vi "filter_logic_delays_test.vi"() -> ()   [LabVIEW 2015]
uses:
  <vilib>/Platform/TimedLoop/XDataNode/timing_clust.ctl
  <vilib>/Platform/TimedLoop/XDataNode/nitl_modes.ctl
  <vilib>/Platform/TimedLoop/XDataNode/wakeup.ctl
  <vilib>/rvi/Emulation/niFpgaGetClockAttributes.vi
  <vilib>/rvi/Emulation/niFpgaSctlEmulationGetInTimedLoop.vi
  <vilib>/rvi/Emulation/niFpgaEmulationReportErrorSimple.vi
  <vilib>/rvi/Emulation/niFpgaProcessEmulError.vi
  <vilib>/rvi/eio/common/nirviEmuTemplateMethod_errors.vi
  <vilib>/rvi/Emulation/niFpgaCriticalErrorInLSC.vi
  <vilib>/eio/EIONode/EIONode.xnode
  <vilib>/Platform/TimedLoop/XDataNode/XDataNode.xnode
  <vilib>/Platform/TimedLoop/XDataNode/XDNodeRunTimeDep.lvlib
panel:
  in  "One Shot":bool
  in  "High Charge Limit":i16
  in  "Low Charge Limit":i16
  in  "High Velocity Count":i32
  in  "Low Velocity Count":i32
  in  "High Mass Limit":i64
  in  "Low Mass Limit":i64
  in  "Mult1":fxp<+,16,7>
  out "Plates":bool
  out "Delay":bool
  out "Armed":bool
  out "Del Armed":bool
  in  "Reset One Shot":bool
  in  "Filter threshold 1":i32=1000
  in  "Filter threshold 2":i32=1000
  in  "Filter threshold 3":i32=1000
  in  "Filter threshold 4":i32=1000
  in  "Filter threshold 5":i32=1000
  in  "Filter threshold 6":i32=1000
  in  "Filter threshold 7":i32=1000
  out "Detector 1 Correlation 2":i16
  out "Detector 1 Correlation 1":i16
  out "Detector 3 Correlation 1":i16
  out "Detector 3 Correlation 2":i16
  out "Detector 1 Correlation 3":i16
  out "Detector 1 Correlation 4":i16
  out "Detector 3 Correlation 3":i16
  out "Detector 1 Correlation 5":i16
  out "Detector 3 Correlation 4":i16
  out "Detector 1 Correlation 6":i16
  out "Detector 3 Correlation 5":i16
  out "Detector 1 Correlation 7":i16
  out "Detector 3 Correlation 6":i16
  out "Detector 3 Correlation 7":i16
  out "IO Module\\AI 0":i16
  out "IO Module\\AI 1":i16
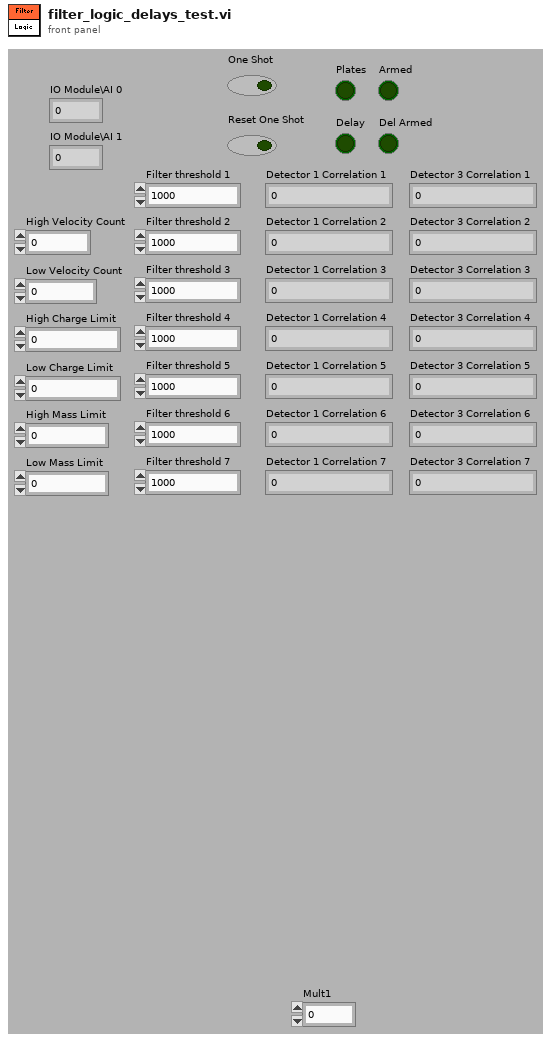
[diagram p1: front panel]
types:
  T1 = typedef "XDNodeRunTimeDep.lvlib/timing_clust.ctl" = cluster{"Expected End [f-1]":u64, "Actual End [f-1]":u64, "Finished Late? [f-1]":bool, "Expected End [i-1]":u64, "Actual End [i-1]":u64, "Finished Late? [i-1]":bool, "Expected Start [i]":u64, "Actual Start [i]":u64, "Expected Start [f]":u64, "Actual Start [f]":u64, "Source Name":string, "Structure Name":string, "Period":i64, "Deadline":i64, "Offset":i64, "Start":i64, "Priority":i32, "Timeout":i32, "Mode":T2, "Wakeup Reason":T3, "Error":errorcluster, "Source Type":string, "Secondary Source Type":string, "Global End Time":u64, "Global Start Time":u64, "Frame Duration":u64, "Iteration Duration":u64, "Assigned CPU":i32, "I/O Scan Engine Mode":u32}
  T2 = typedef "XDNodeRunTimeDep.lvlib/nitl_modes.ctl" = enum32{"No Change", "Process missed periods, maintain original phase", "Discard missed periods, maintain original phase", "Process missed periods, ignore original phase", "Discard missed periods, ignore original phase"}
  T3 = typedef "XDNodeRunTimeDep.lvlib/wakeup.ctl" = enum32{"Normal", "Aborted", "Asynchronous wakeup", "Timing source error", "Timed loop error", "Timeout"}
  T4 = typedef "Limits.ctl" = cluster{"High Charge Limit":i16, "Low Charge Limit":i16, "Time Out Limit":i32, "High Velocity Count":i32, "Low Velocity Count":i32, "Sampling Rate":fxp<+,30,25>, "High Mass Limit":i64, "Low Mass Limit":i64}
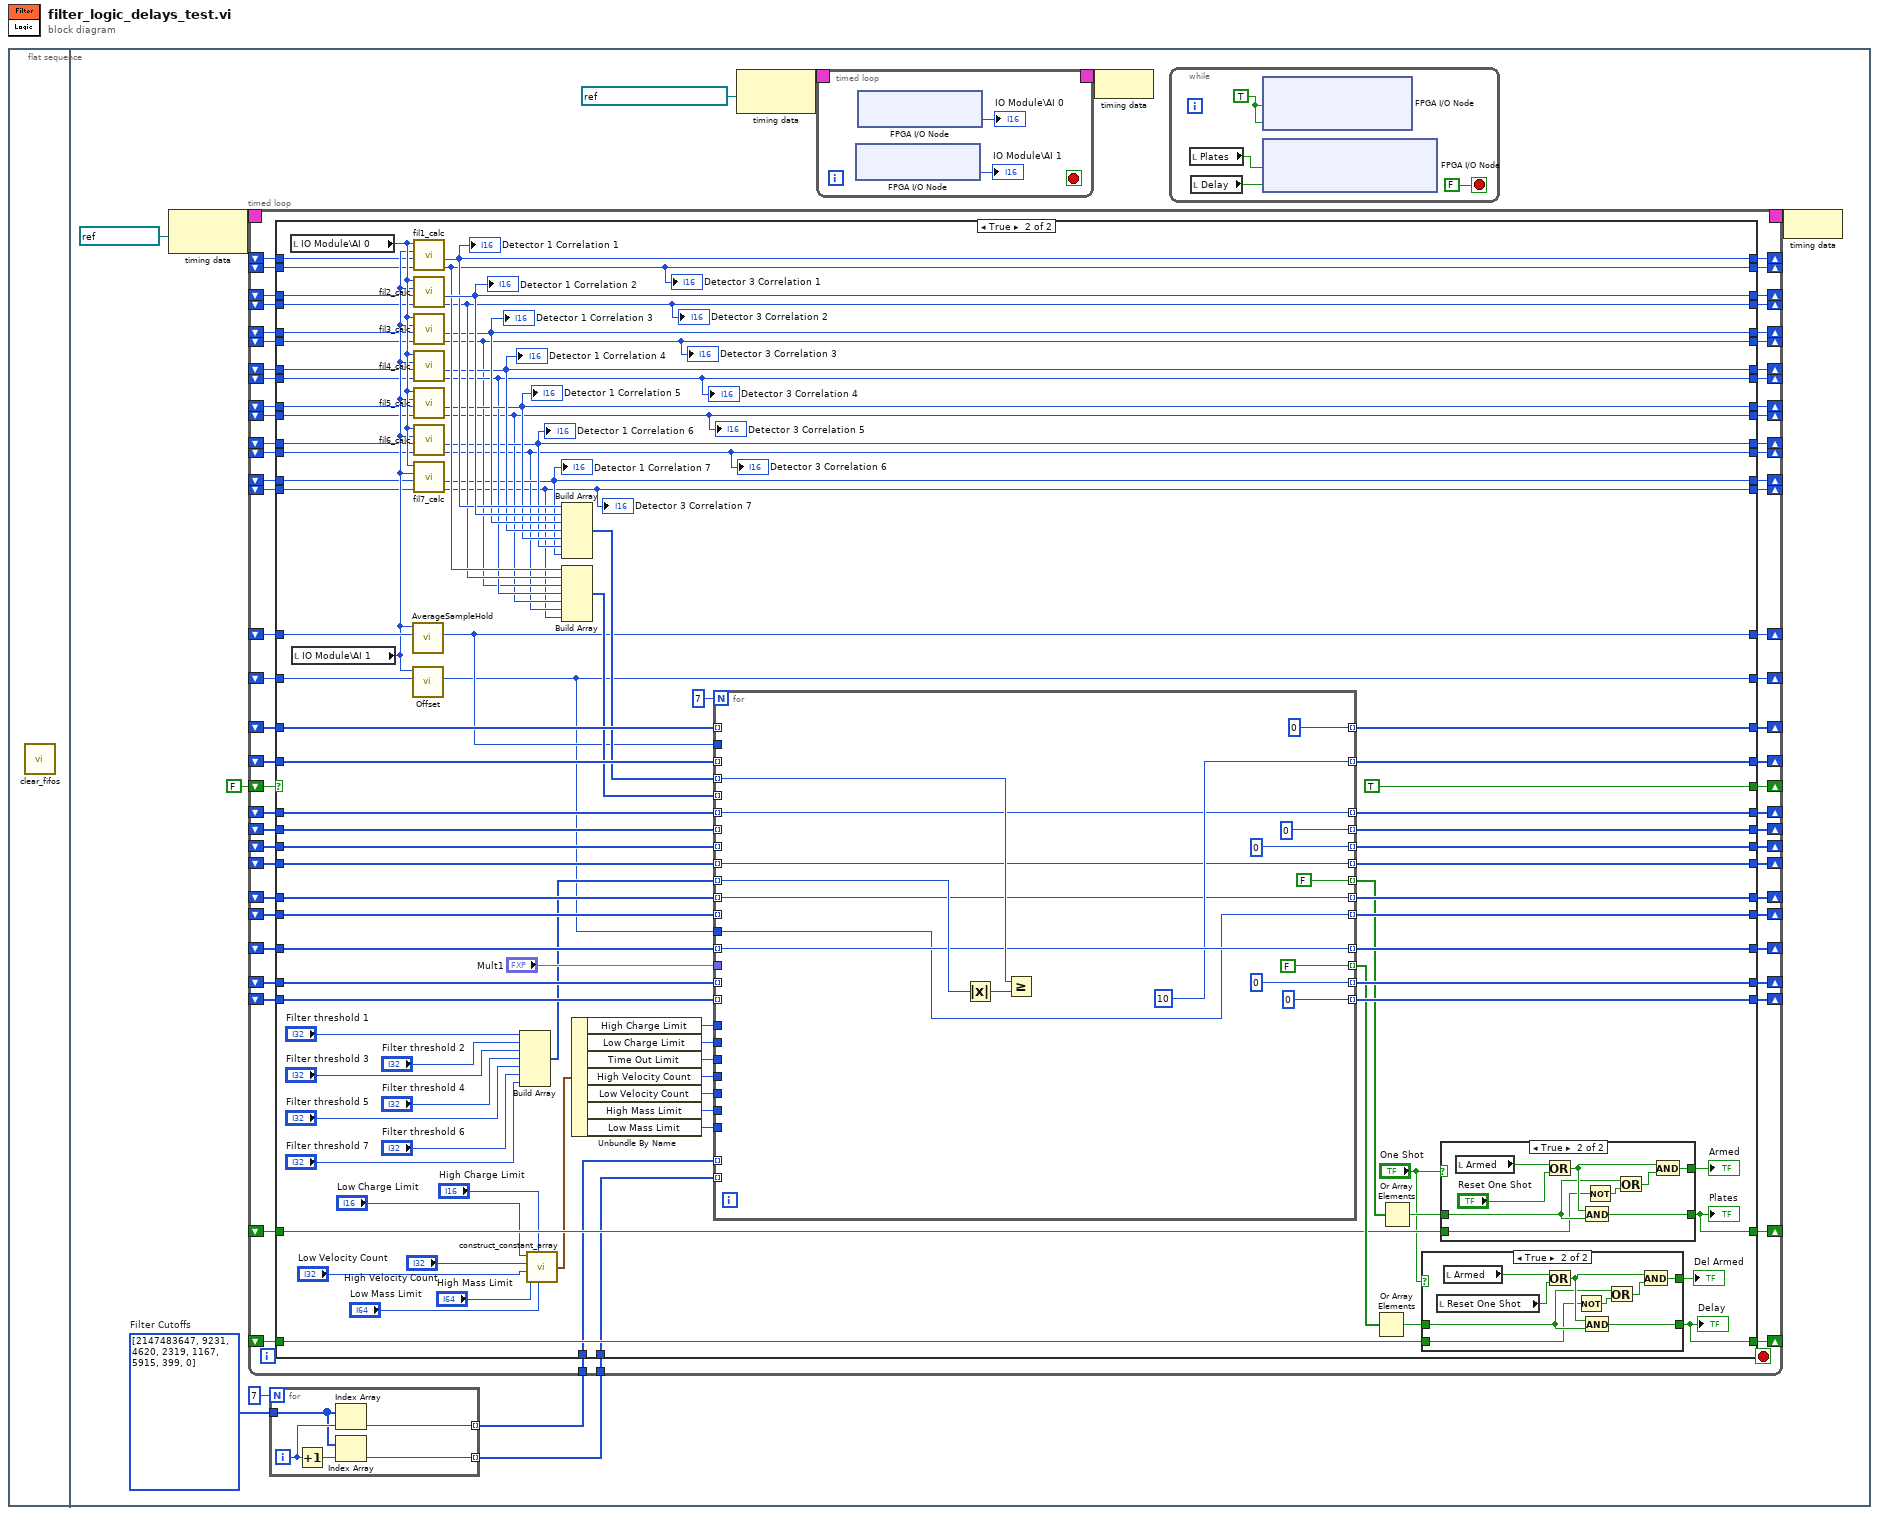
[diagram p0: block diagram]
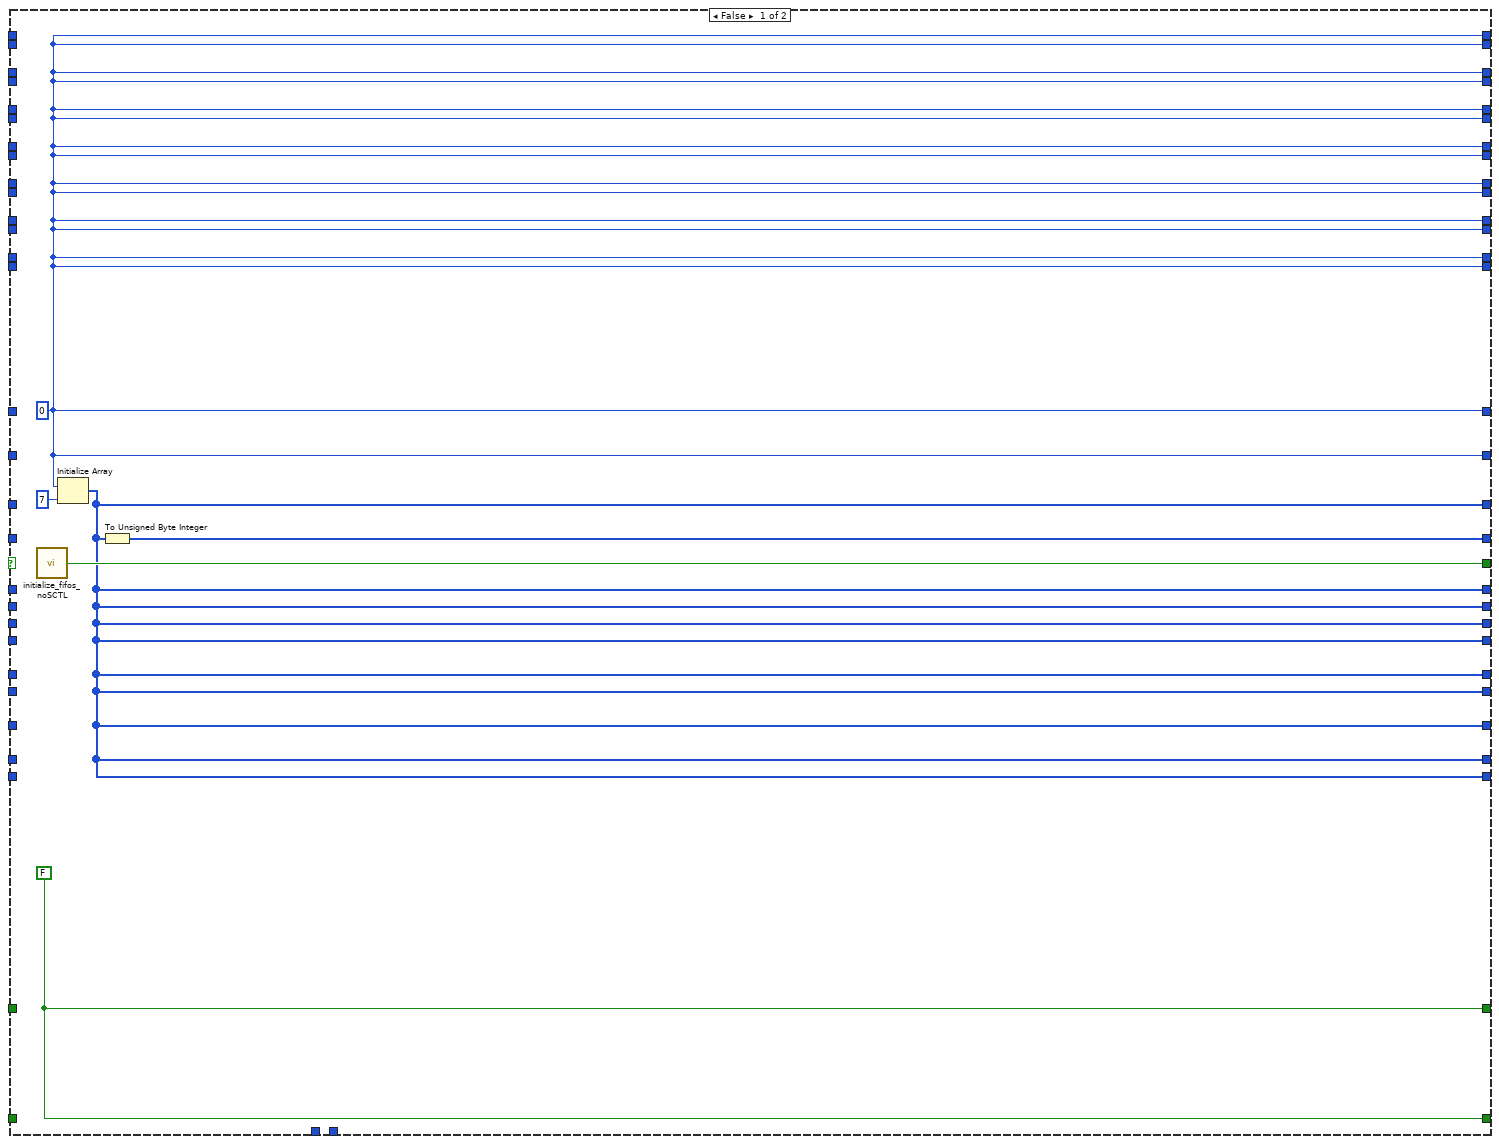
[diagram p2: hidden frame]
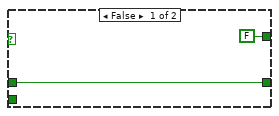
[diagram p3: hidden frame]
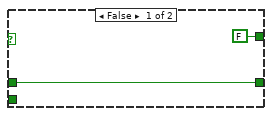
[diagram p4: hidden frame]
diagram:
  n1 = flat-sequence {
    frame #0 {
      n2 = call "clear_fifos.vi"() -> ()  [unwired: 1 in]
    }
    frame #1 {
      w3 = i32[] [2147483647, 9231, 4620, 2319, 1167, 5915, 399, 0]  # Filter Cutoffs
      n3 = node-c288(refnum<k21> "26.67MHz" ("Source Name")) -> (w11:T1)
      n4 = for {
        N: 7 -> [_]
        tunnel: w3 -> [w14]
        tunnel: [w13] -> w2 mode=indexing
        tunnel: [w12] -> w1 mode=indexing
        i -> [w16]
        n5 = Increment(x=w16) -> (x+1=w15:i32)
        n6 = Index Array(array=w14, index=w16) -> (element=w13:i32)
        n7 = Index Array(array=w14, index=w15) -> (element=w12:i32)
      }
      n8 = timed-loop {
        timing: w11 -> [_]
        timing-out: [_] -> w10
        shift-right: [w89] -> _
        shift-left: FALSE -> [w90]
        shift-right: [w87] -> _
        shift-left: _ -> [w88]
        shift-right: [w85] -> _
        shift-left: _ -> [w86]
        shift-right: [w83] -> _
        shift-left: _ -> [w84]
        shift-right: [w69] -> _
        shift-left: _ -> [w82]
        shift-right: [w80] -> _
        shift-left: _ -> [w81]
        shift-right: [w78] -> _
        shift-left: _ -> [w79]
        shift-right: [w68] -> _
        shift-left: _ -> [w77]
        shift-right: [w67] -> _
        shift-left: _ -> [w76]
        shift-right: [w63] -> _
        shift-left: _ -> [w75]
        shift-right: [w73] -> _
        shift-left: _ -> [w74]
        shift-right: [w66] -> _
        shift-left: _ -> [w72]
        shift-right: [w65] -> _
        shift-left: _ -> [w71]
        shift-right: [w64] -> _
        shift-left: _ -> [w70]
        shift-right: [w62] -> _
        shift-left: _ -> [w61]
        shift-right: [w59] -> _
        shift-left: _ -> [w60]
        shift-right: [w58] -> _
        shift-left: _ -> [w57]
        shift-right: [w56] -> _
        shift-left: _ -> [w55]
        shift-right: [w54] -> _
        shift-left: _ -> [w50]
        shift-right: [w53] -> _
        shift-left: _ -> [w49]
        shift-right: [w52] -> _
        shift-left: _ -> [w48]
        shift-right: [w51] -> _
        shift-left: _ -> [w47]
        shift-right: [w46] -> _
        shift-left: _ -> [w38]
        shift-right: [w45] -> _
        shift-left: _ -> [w37]
        shift-right: [w44] -> _
        shift-left: _ -> [w36]
        shift-right: [w43] -> _
        shift-left: _ -> [w31]
        shift-right: [w42] -> _
        shift-left: _ -> [w35]
        shift-right: [w41] -> _
        shift-left: _ -> [w32]
        shift-right: [w40] -> _
        shift-left: _ -> [w34]
        shift-right: [w39] -> _
        shift-left: _ -> [w33]
        tunnel: w2 -> [w30]
        tunnel: w1 -> [w29]
        stop <- _ stop-if-true
        n9 = case shown="True" w90 {
          tunnel: [w96 TRUE] -> w89
          tunnel: w88 -> [_ w191]
          tunnel: [w93 w190] -> w87
          tunnel: w86 -> [_ w189]
          tunnel: [w91 w123] -> w85
          tunnel: w84 -> [_ w188]
          tunnel: [w94 w187] -> w83
          tunnel: w82 -> [_ w186]
          tunnel: w81 -> [_ w185]
          tunnel: [w93 w184] -> w80
          tunnel: w79 -> [_ w183]
          tunnel: [w93 w182] -> w78
          tunnel: w77 -> [_ w181]
          tunnel: w76 -> [_ w180]
          tunnel: w75 -> [_ w179]
          tunnel: w74 -> [_ w178]
          tunnel: [w91 w122] -> w73
          tunnel: w72 -> [_ w177]
          tunnel: w71 -> [_ w176]
          tunnel: w70 -> [_ w175]
          tunnel: [w93 w174] -> w69
          tunnel: [w93 w173] -> w68
          tunnel: [w93 w172] -> w67
          tunnel: [w93 w171] -> w66
          tunnel: [w93 w170] -> w65
          tunnel: [w93 w169] -> w64
          tunnel: [w93 w168] -> w63
          tunnel: [w95 w162] -> w62
          tunnel: w61 -> [_ w163]
          tunnel: w60 -> [_ w159]
          tunnel: [w95 w158] -> w59
          tunnel: [w91 w108] -> w58
          tunnel: w57 -> [_ w137]
          tunnel: [w91 w110] -> w56
          tunnel: w55 -> [_ w136]
          tunnel: [w91 w109] -> w54
          tunnel: [w91 w112] -> w53
          tunnel: [w91 w111] -> w52
          tunnel: [w91 w115] -> w51
          tunnel: w50 -> [_ w135]
          tunnel: w49 -> [_ w134]
          tunnel: w48 -> [_ w133]
          tunnel: w47 -> [_ w132]
          tunnel: [w91 w114] -> w46
          tunnel: [w91 w116] -> w45
          tunnel: [w91 w113] -> w44
          tunnel: [w91 w117] -> w43
          tunnel: [w91 w118] -> w42
          tunnel: [w91 w121] -> w41
          tunnel: [w91 w119] -> w40
          tunnel: [w91 w120] -> w39
          tunnel: w38 -> [_ w131]
          tunnel: w37 -> [_ w130]
          tunnel: w36 -> [_ w129]
          tunnel: w35 -> [_ w128]
          tunnel: w34 -> [_ w127]
          tunnel: w33 -> [_ w126]
          tunnel: w32 -> [_ w125]
          tunnel: w31 -> [_ w124]
          tunnel: w30 -> [_ w107]
          tunnel: w29 -> [_ w106]
          frame False {
            w95 = FALSE
            w91 = i16 0 ("Output New Average")
            n10 = call "initialize_fifos_noSCTL.vi"() -> ("Output State"=w96:bool)
            n11 = Initialize Array(w91, 7 ("dimension size")) -> (w93:i16[])
            n12 = To Unsigned Byte Integer(number=w93) -> (unsigned 8bit integer=w94:u8[])
          }
          frame True {
            n13 = local read "IO Module\\AI 0"() -> (w149:i16)
            n14 = local read "IO Module\\AI 1"() -> (w148:i16)
            n15 = call "AverageSampleHold.vi"("Previous Average"=w189, "Input Value"=w148) -> ("Output New Average"=w123:i16)  [unwired: 9 in]
            n16 = call "Offset.vi"("Previous Average"=w178, "Input Value"=w148) -> ("Output New Average"=w122:i16)  [unwired: 9 in]
            n17 = call "fil1_calc.vi"("Detector 3 Correlation In"=w127, "Detector 1 Correlation In"=w126, "AI1"=w148, "AI0"=w149) -> ("Detector 3 Correlation Out"=w119:i16, "Detector 1 Correlation Out"=w120:i16)  [unwired: 4 in]
            "Detector 1 Correlation 1" <- w120
            "Detector 3 Correlation 1" <- w119
            n18 = call "fil2_calc.vi"("Detector 3 Correlation In"=w128, "Detector 1 Correlation In"=w125, "AI1"=w148, "AI0"=w149) -> ("Detector 3 Correlation Out"=w118:i16, "Detector 1 Correlation Out"=w121:i16)  [unwired: 4 in]
            "Detector 1 Correlation 2" <- w121
            "Detector 3 Correlation 2" <- w118
            n19 = call "fil3_calc.vi"("Detector 3 Correlation In"=w129, "Detector 1 Correlation In"=w124, "AI1"=w148, "AI0"=w149) -> ("Detector 3 Correlation Out"=w113:i16, "Detector 1 Correlation Out"=w117:i16)  [unwired: 4 in]
            "Detector 1 Correlation 3" <- w117
            "Detector 3 Correlation 3" <- w113
            n20 = call "fil4_calc.vi"("Detector 3 Correlation In"=w131, "Detector 1 Correlation In"=w130, "AI1"=w148, "AI0"=w149) -> ("Detector 3 Correlation Out"=w114:i16, "Detector 1 Correlation Out"=w116:i16)  [unwired: 4 in]
            "Detector 1 Correlation 4" <- w116
            "Detector 3 Correlation 4" <- w114
            n21 = call "fil5_calc.vi"("Detector 3 Correlation In"=w133, "Detector 1 Correlation In"=w132, "AI1"=w148, "AI0"=w149) -> ("Detector 3 Correlation Out"=w111:i16, "Detector 1 Correlation Out"=w115:i16)  [unwired: 4 in]
            "Detector 1 Correlation 5" <- w115
            "Detector 3 Correlation 5" <- w111
            n22 = call "fil6_calc.vi"("Detector 3 Correlation In"=w135, "Detector 1 Correlation In"=w134, "AI1"=w148, "AI0"=w149) -> ("Detector 3 Correlation Out"=w109:i16, "Detector 1 Correlation Out"=w112:i16)  [unwired: 4 in]
            "Detector 1 Correlation 6" <- w112
            "Detector 3 Correlation 6" <- w109
            n23 = call "fil7_calc.vi"("Detector 3 Correlation In"=w137, "Detector 1 Correlation In"=w136, "AI1"=w148, "AI0"=w149) -> ("Detector 3 Correlation Out"=w108:i16, "Detector 1 Correlation Out"=w110:i16)  [unwired: 4 in]
            "Detector 1 Correlation 7" <- w110
            "Detector 3 Correlation 7" <- w108
            n24 = Build Array("Filter threshold 1", "Filter threshold 2", "Filter threshold 3", "Filter threshold 4", "Filter threshold 5", "Filter threshold 6", "Filter threshold 7") -> (w138:i32[])
            n25 = call "construct_constant_array.vi"("Low Mass Limit"="Low Mass Limit", "High Charge Limit"="High Charge Limit", "High Mass Limit"="High Mass Limit", "Low Velocity Count"="Low Velocity Count", "High Velocity Count"="High Velocity Count", "Low Charge Limit"="Low Charge Limit") -> ("Limits"=w105:T4)
            n26 = Build Array(w120, w121, w117, w116, w115, w112, w110) -> (w147:i16[])
            n27 = Build Array(w119, w118, w113, w114, w111, w109, w108) -> (w146:i16[])
            n28 = Unbundle By Name(w105) -> ("High Charge Limit"=w98:i16, "Low Charge Limit"=w99:i16, "Time Out Limit"=w100:i32, "High Velocity Count"=w101:i32, "Low Velocity Count"=w102:i32, "High Mass Limit"=w103:i64, "Low Mass Limit"=w104:i64)
            n29 = for {
              N: 7 -> [_]
              tunnel: w147 -> [w230] mode=indexing
              tunnel: w146 -> [_] mode=indexing
              tunnel: w191 -> [_] mode=indexing
              tunnel: [0 ("Old Average In")] -> w190 mode=indexing
              tunnel: w188 -> [_] mode=indexing
              tunnel: [u8 10] -> w187 mode=indexing
              tunnel: w186 -> [w225] mode=indexing
              tunnel: w185 -> [_] mode=indexing
              tunnel: [0] -> w184 mode=indexing
              tunnel: w183 -> [_] mode=indexing
              tunnel: [u16 0] -> w182 mode=indexing
              tunnel: w181 -> [_] mode=indexing
              tunnel: w180 -> [_] mode=indexing
              tunnel: w179 -> [w228] mode=indexing
              tunnel: w177 -> [w222] mode=indexing
              tunnel: w138 -> [w229] mode=indexing
              tunnel: w176 -> [w219] mode=indexing
              tunnel: w175 -> [_] mode=indexing
              tunnel: [w225] -> w174 mode=indexing
              tunnel: [0] -> w173 mode=indexing
              tunnel: [u32 0] -> w172 mode=indexing
              tunnel: [w222] -> w171 mode=indexing
              tunnel: [w219] -> w170 mode=indexing
              tunnel: [w218] -> w169 mode=indexing
              tunnel: [w228] -> w168 mode=indexing
              tunnel: [FALSE] -> w167 mode=indexing
              tunnel: [FALSE] -> w166 mode=indexing
              tunnel: "Mult1" -> [_]
              tunnel: w123 -> [_]
              tunnel: w122 -> [w218]
              tunnel: w107 -> [_] mode=indexing
              tunnel: w106 -> [_] mode=indexing
              tunnel: w104 -> [_]
              tunnel: w103 -> [_]
              tunnel: w102 -> [_]
              tunnel: w101 -> [_]
              tunnel: w100 -> [_]
              tunnel: w99 -> [_]
              tunnel: w98 -> [_]
              n30 = Absolute Value(x=w229) -> (abs(x)=w215:i32)
              n31 = Greater Or Equal?(x=w230, y=w215) -> ()  [unwired: 1 out]
            }
            n32 = Or Array Elements(Boolean array=w166) -> (logical OR=w161:bool)
            n33 = Or Array Elements(Boolean array=w167) -> (logical OR=w165:bool)
            n34 = case shown="True" "One Shot" {
              tunnel: [w194 w200] -> w158
              tunnel: w161 -> [w194 w197]
              tunnel: [FALSE w202] -> w157
              tunnel: w159 -> [_ w196]
              frame False {
              }
              frame True {
                n35 = local read "Reset One Shot"() -> (w195:bool)
                n36 = local read "Armed"() -> (w203:bool)
                n37 = Or(x=w203, y=w195) -> (x .or. y?=w201:bool)
                n38 = Not(x=w196) -> (.not. x?=w198:bool)
                n39 = And(x=w201, y=w197) -> (x .and. y?=w200:bool)
                n40 = Or(x=w197, y=w198) -> (x .or. y?=w199:bool)
                n41 = And(x=w201, y=w199) -> (x .and. y?=w202:bool)
              }
            }
            "Delay" <- w158
            "Del Armed" <- w157
            n42 = case shown="True" "One Shot" {
              tunnel: [w205 w210] -> w162
              tunnel: w165 -> [w205 w207]
              tunnel: [FALSE w212] -> w164
              tunnel: w163 -> [_ w206]
              frame False {
              }
              frame True {
                n43 = local read "Armed"() -> (w214:bool)
                n44 = Or(x=w214, y="Reset One Shot") -> (x .or. y?=w211:bool)
                n45 = And(x=w211, y=w207) -> (x .and. y?=w210:bool)
                n46 = Not(x=w206) -> (.not. x?=w208:bool)
                n47 = Or(x=w207, y=w208) -> (x .or. y?=w209:bool)
                n48 = And(x=w211, y=w209) -> (x .and. y?=w212:bool)
              }
            }
            "Plates" <- w162
            "Armed" <- w164
          }
        }
      }
      n49 = node-c288(refnum<k21> "IO Module\\Data Clock" ("Source Name")) -> (w8:T1)
      n50 = timed-loop {
        timing: w8 -> [_]
        timing-out: [_] -> w7
        stop <- _ stop-if-true
        n51 = xnode "FPGA I/O Node"() -> ("IO Module\\AI 1"=→"IO Module\\AI 1":i16)  [unwired: 1 in, 1 out]
        n52 = xnode "FPGA I/O Node"() -> ("IO Module\\AI 0"=→"IO Module\\AI 0":i16)  [unwired: 1 in, 1 out]
      }
      n53 = node-c288(w7) -> ()
      n54 = while {
        stop <- FALSE stop-if-true
        w28 = TRUE ("IO Module\\PFI Enable")
        n55 = local read "Plates"() -> (w26:bool)
        n56 = local read "Delay"() -> (w25:bool)
        n57 = xnode "FPGA I/O Node"("IO Module\\PFI 0 WE"=w28, "IO Module\\PFI 1 WE"=w28) -> ()  [unwired: 2 in, 2 out]
        n58 = xnode "FPGA I/O Node"("IO Module\\PFI 0 Wr Data"=w26, "IO Module\\PFI 1 Wr Data"=w25) -> ()  [unwired: 2 in, 2 out]
      }
      n59 = node-c288(w10) -> ()
    }
  }
